vi "main.vi"   [LabVIEW 2023]
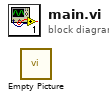
[diagram p0: block diagram]
diagram:
  n1 = call "Empty Picture"() -> ()  [unwired: 1 out]
